vi "Read.vi"(8 "error in (no error)":errorcluster, 9 "Starting independent variables":dbl[](array[numeric]), 10 "Current independent variables":dbl[](array[numeric]), 11 "Two lockins reader in":refnum<class "Two lockins reader.lvclass">) -> (0 "error out":errorcluster, 2 "Data Channels":T1, 3 "Two lockins reader out":refnum<class "Two lockins reader.lvclass">)   [LabVIEW 2017, in "Two lockins reader.lvclass"]
doc: "Prepare for read, wait the time delay, and take data from up to 4 channels."
uses:
  Two lockins reader.lvclass
  Instruments/Utility Classes/Readable/Data Channels.ctl
  Instruments/Utility Classes/Readable/Data Channel.ctl
  Instruments/Utility Classes/Readable/Data Point.ctl
  Instruments/Utility Classes/Readable/Time.ctl
  Instruments/Utility Classes/Readable/X.ctl
  Two lockins reader.lvclass/Two lockins reader.ctl
  Reader/Reader.lvclass
  Instruments/Lockin/Lockin SR830.lvclass
  Instruments/Utility Classes/Readable/Readable.lvclass
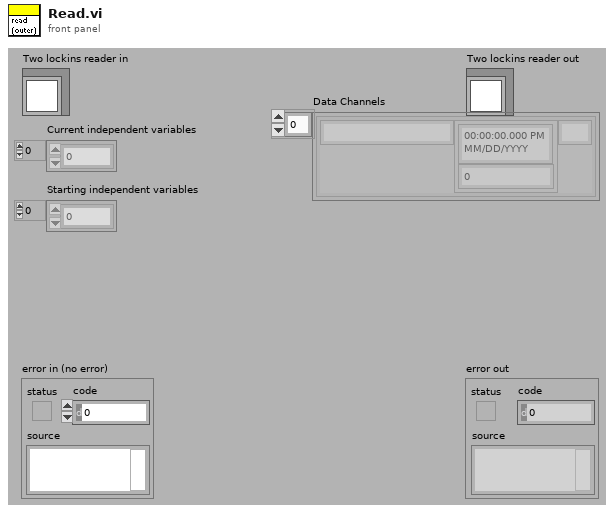
[diagram p1: front panel]
types:
  T1 = typedef "Readable.lvclass/Data Channels.ctl" = T2[]
  T2 = typedef "Readable.lvclass/Data Channel.ctl" = cluster{"Name":string, "Data Point":T3, "Unit":string}
  T3 = typedef "Readable.lvclass/Data Point.ctl" = cluster{"t":T4, "x":T5}
  T4 = typedef "Readable.lvclass/Time.ctl" = timestamp
  T5 = typedef "Readable.lvclass/X.ctl" = dbl
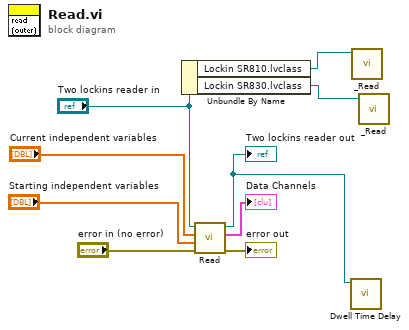
[diagram p0: block diagram]
diagram:
  n1 = Unbundle By Name("Two lockins reader in") -> ("Lockin SR810.lvclass"=w3:refnum<class "Lockin SR830.lvclass">, "Lockin SR830.lvclass"=w2:refnum<class "Lockin SR830.lvclass">)
  n2 = call-parent "Read.vi"("error in (no error)"="error in (no error)", "Starting independent variables"="Starting independent variables", "Current independent variables"="Current independent variables", "Reader in"="Two lockins reader in") -> ("error out"=→"error out":errorcluster, "Data Channels"=→"Data Channels":T1, "Reader out"=w1:refnum<class "Two lockins reader.lvclass">)  [unwired: 5 in]
  "Two lockins reader out" <- w1
  n3 = call-dynamic "Dwell Time Delay.vi"("Reader in"=w1) -> ()  [unwired: 1 in, 10 out]
  n4 = call-dynamic "_Read.vi"("Lockin SR830 in"=w3) -> ()  [unwired: 8 in, 3 out]
  n5 = call-dynamic "_Read.vi"("Lockin SR830 in"=w2) -> ()  [unwired: 8 in, 3 out]
